vi "Get Serial (uSMC).vi"(8 "error in (no error)":errorcluster, 9 "Index":i32, 11 "Visa array in":refnum<visa-resource-name>[](array[refnum])) -> (0 "error out":errorcluster, 1 "Serial Number":string, 3 "Visa array out":refnum<visa-resource-name>[](array[refnum]))   [LabVIEW 2010, in "SignalWriterMH110203USBStepperMotor.lvclass"]
uses:
  SignalWriterMH110203USBStepperMotor.lvclass
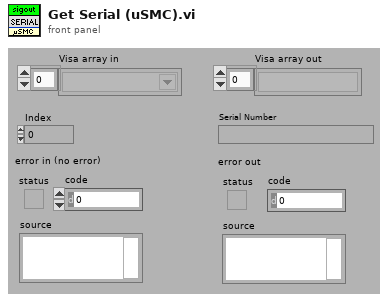
[diagram p1: front panel]
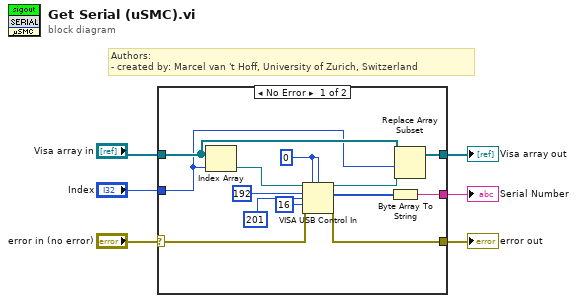
[diagram p0: block diagram]
diagram:
  # "Authors: \n- created by: Marcel van 't Hoff, University of Zurich, Switzerland"
  n1 = case shown="No Error" "error in (no error)" {
    selector: "error in (no error)" -> [w7 w21]
    tunnel: [w19 w21] -> w6
    tunnel: [w13 _] -> w5
    tunnel: "Visa array in" -> [w11 w20]
    tunnel: "Index" -> [w9 _]
    tunnel: [w8 w20] -> w2
    frame No Error {
      w15 = u16 0 ("value (0)")
      n2 = Index Array(array=w11, index=w9) -> (element=w12:refnum<visa-resource-name>)
      n3 = VISA USB Control In(0:w12, 1:w15, 2:w15, 5:i16 192 ("request type"), 7:i16 201 ("request"), 9:u16 16 ("length (0)"), 11:w7) -> (4:w10:refnum<visa-resource-name>, 6:w14:u8[], 15:w19:errorcluster)
      n4 = Byte Array To String(unsigned byte array=w14) -> (string=w13:string)
      n5 = Replace Array Subset(array=w11, new element=w10, index=w9) -> (w8:refnum<visa-resource-name>[])
    }
    frame Error {
    }
  }
  "error out" <- w6
  "Serial Number" <- w5
  "Visa array out" <- w2
